vi "TM submodule LSC218.vi"(10 "name (Tmp_M)":string="Tmp_M" caption="Module name", 11 "Super module":T2) -> (0 "Error Out":errorcluster)   [LabVIEW 2021, in "Temperature monitor.lvlib"]
doc: "Magnet module controls: power supply unit (PSU/SMS) and temperature monitor (TM/LSC218).\nPSU controls mainly: switch heater and ramping of current which runs throught coil.\nTM controls temperature of switch, coil and cryostat.\nMessage for magnet is a cluster that contains: {(enum) Command , (variant) Data}\nFor simplifieing of documentation, the Command is noted as a name of instruction, and Data is represented by a requered datatype (mostly cluster) name.\nCommands:\nInitialize(Magnet Config Constants) - Sugesstion: Load configuration constants from configuration file.\nSet field (Set field{B, R, cr}) - B-field[T], R-ramp[A/s], cr - custom ramp[bool].\nSwitch mode(mode) - to persistant, or to ramping.\nBlackout() - undone functionality of emergency deenergizing.\nUpdate() - Important! This triggers update of data from instruments. Shoud occure in regular intervals as priority message.\nResponses:\nMagnet initialized ();\nTM revision(temperature monitor revision);\nMagnet init error(error);\nSetting field(Set Field{B, R, cr});\nWarning(string);\nSwitching to(mode);\nUpdate error(error);\nTM update(TM sensors);\nPSU update(PSU data);\nMagnet status();"
uses:
  Temperature monitor.lvlib
  Typedefs/TM_sensors.ctl
  Typedefs/TM_states.ctl
  <userlib>/MatS Libs/MatS Libs.lvlib
  <userlib>/MatS Libs/MatS Mailman/TypeDefs/Mailbox ref.ctl
  Typedefs/TM_status.ctl
  Typedefs/TM_commands.ctl
  <userlib>/MatS Libs/MatS Mailman/TypeDefs/General message.ctl
panel:
  out "Waveform Graph":waveform(dbl)[](graph)
  in  "Disconnect btn":bool
  in  "History s":i32=60 caption="History [s]" min=10 max=3600 step=1
  out "Temperature history":waveform(dbl)[](graph)
  out "Temperature monitor status":T1 caption="Status" {"Last update" format="%<%H:%M:%S\n%y/%m/%d>T"}
  in  "Stop btn":bool
  in  "Connect btn":bool
  out "Temperatures":T3[](array[typedef]) {"Time stamp" format="%<%H:%M:%S\n%Y/%m/%d>T"}
  in  "VISA resource (COM1)":refnum<visa-resource-name>="COM1" caption="Instrument port"
  in  "Update ms":i32=1000
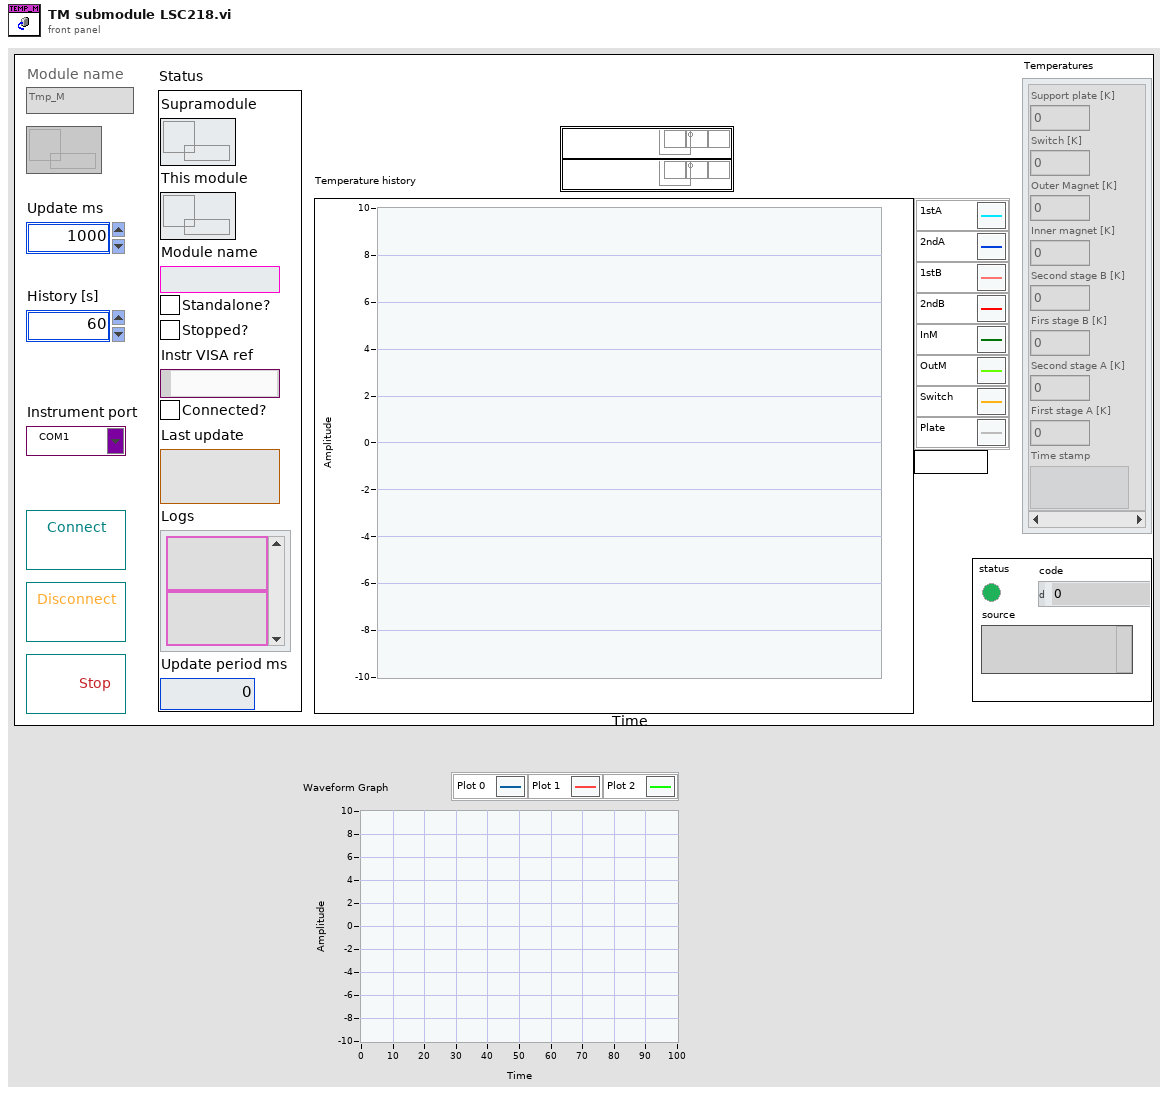
[diagram p1: front panel]
types:
  T1 = typedef "Temperature monitor.lvlib/TM_status.ctl" = cluster{"Supramodule":T2, "This module":T2, "Module name":string, "Standalone?":bool, "Stopped?":bool, "Instr VISA ref":refnum<visa-resource-name>, "Connected?":bool, "Last update":timestamp, "Logs":string[], "Update period ms":u32}
  T2 = typedef "MatS Libs.lvlib/Mailbox ref.ctl" = refnum<queue>
  T3 = typedef "Temperature monitor.lvlib/TM_sensors.ctl" = cluster{"Support plate [K]":dbl, "Switch [K]":dbl, "Outer Magnet [K]":dbl, "Inner magnet [K]":dbl, "Second stage B [K]":dbl, "Firs stage B [K]":dbl, "Second stage A [K]":dbl, "First stage A [K]":dbl, "Time stamp":timestamp}
  T4 = typedef "Temperature monitor.lvlib/TM_states.ctl" = enum16{"Initialize", "Wait for event", "Check message", "Check changes", "End"}
  T5 = enum32{"Bad", "Idle", "Run top level", "Running"}
  T6 = typedef "Temperature monitor.lvlib/TM_commands.ctl" = enum16{"Ignore", "Log", "Connect", "Set timeout", "Update", "Disconnect", "End"}
  T7 = typedef "MatS Libs.lvlib/General message.ctl" = cluster{"Sender":string, "Recipient":string, "Topic":variant, "Content":variant, "Time Stamp":timestamp}
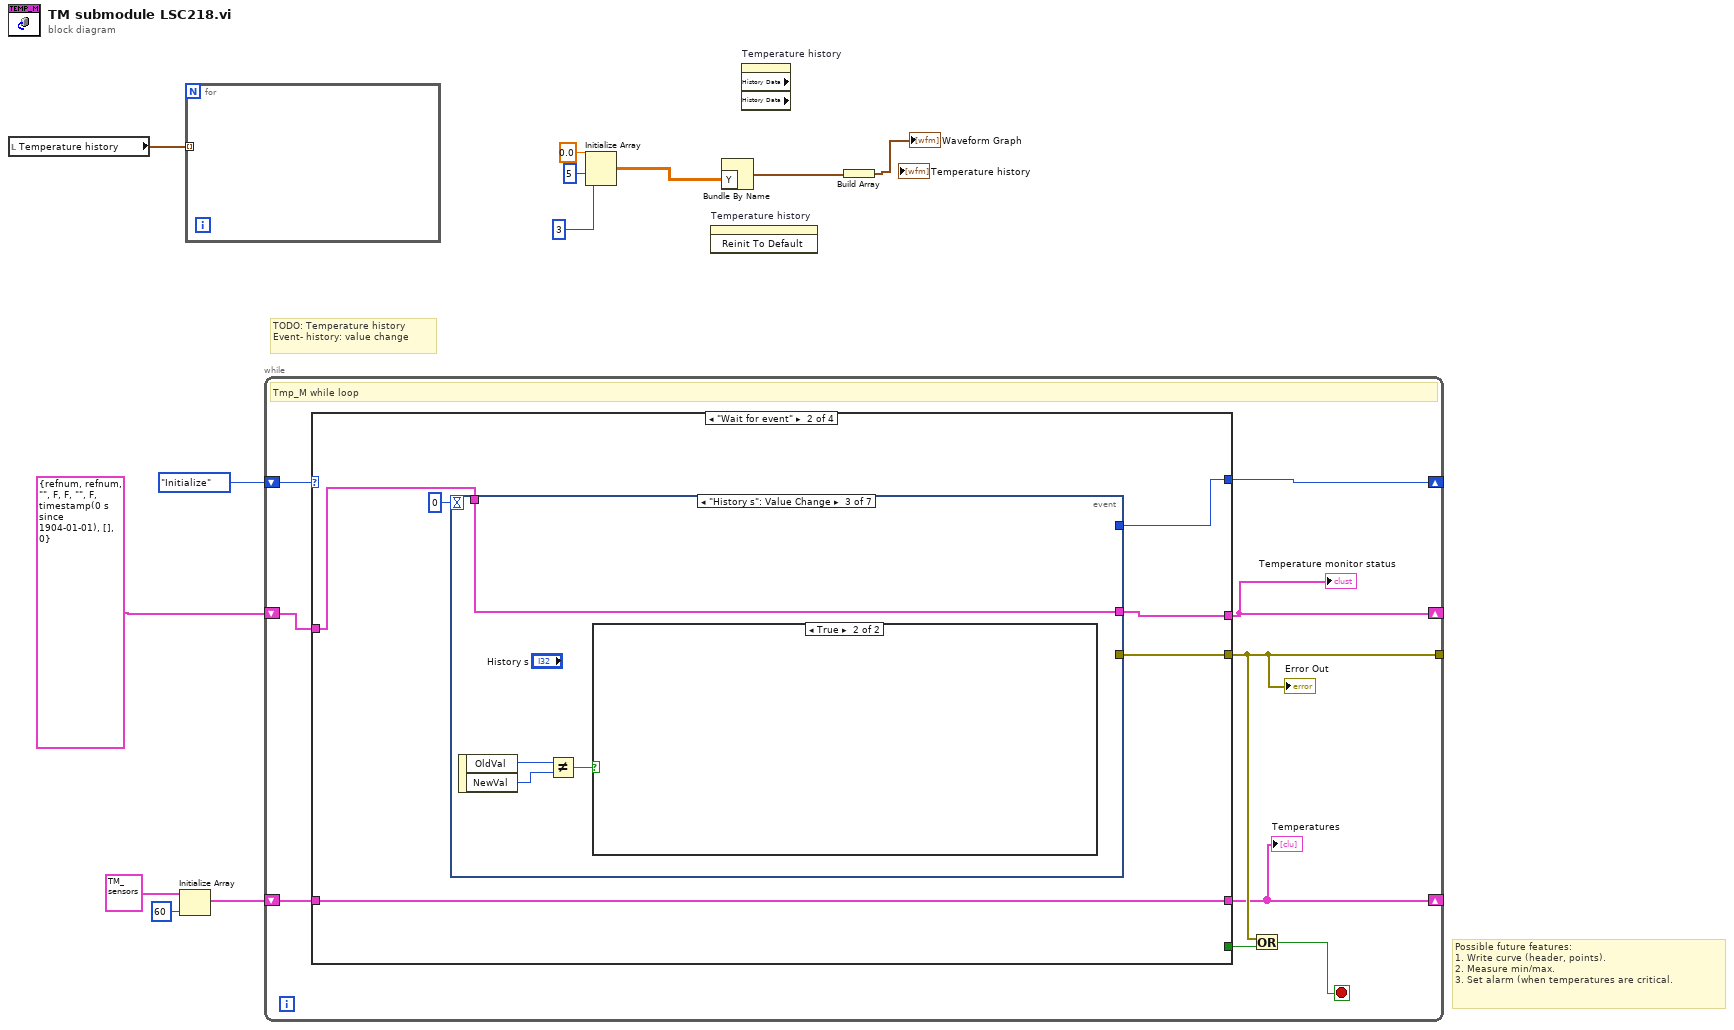
[diagram p0: block diagram]
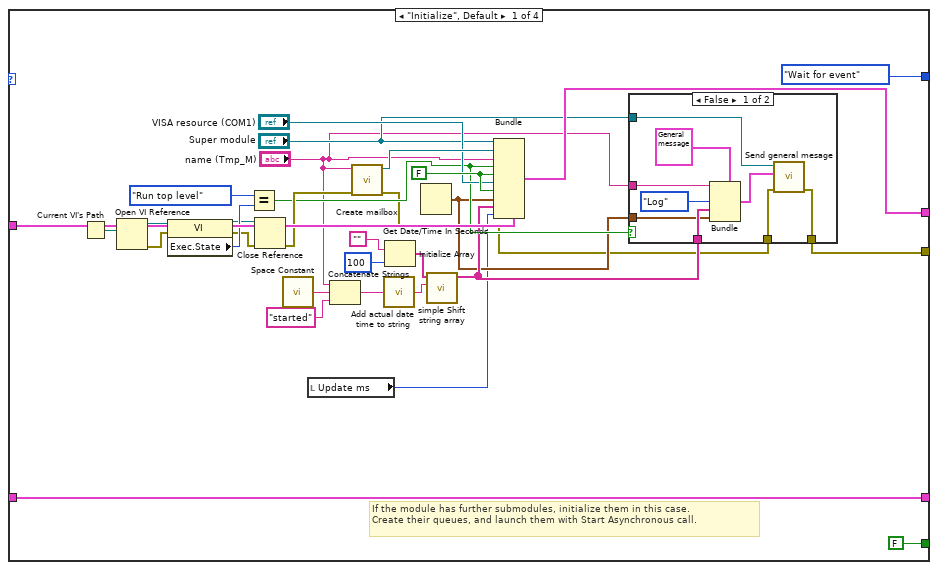
[diagram p2: hidden frame]
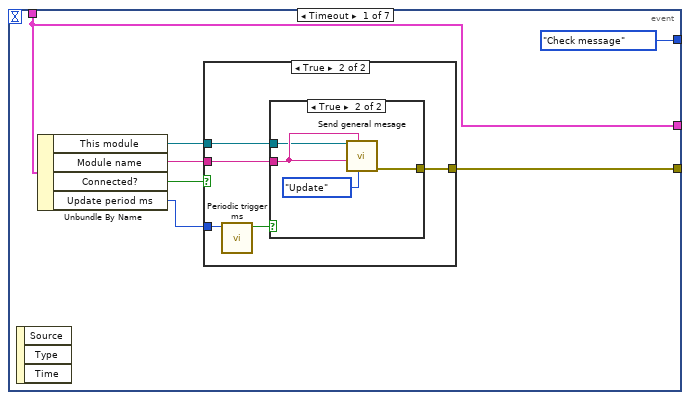
[diagram p4: hidden frame]
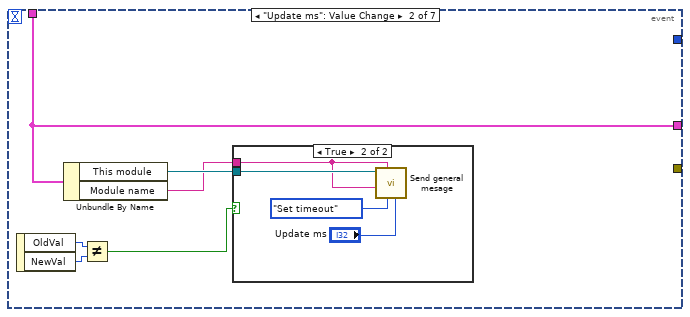
[diagram p7: hidden frame]
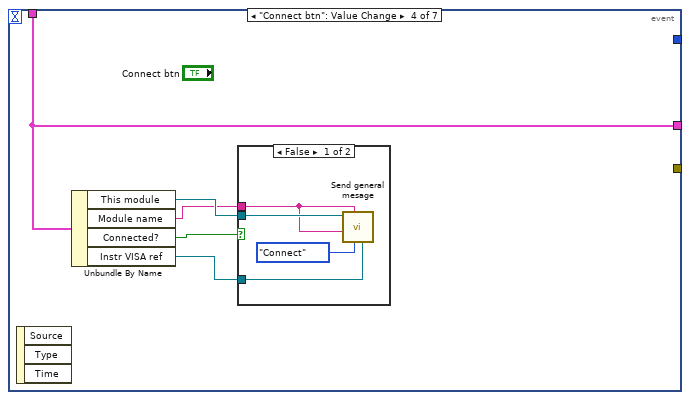
[diagram p10: hidden frame]
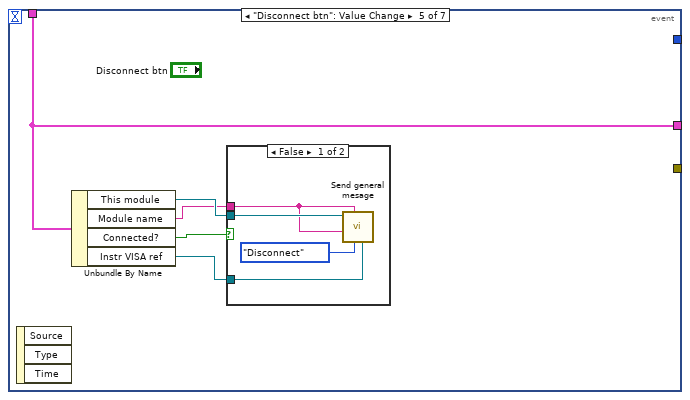
[diagram p12: hidden frame]
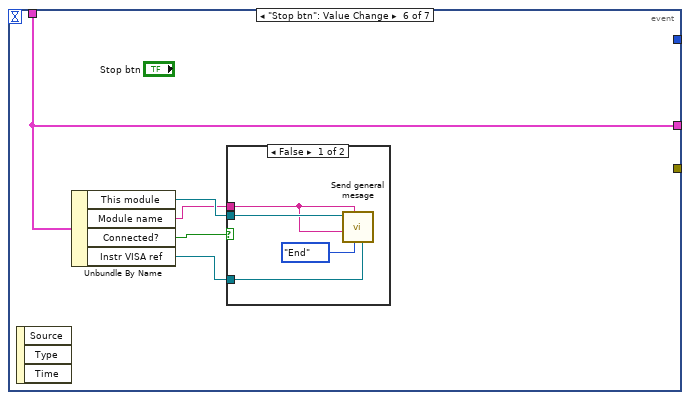
[diagram p14: hidden frame]
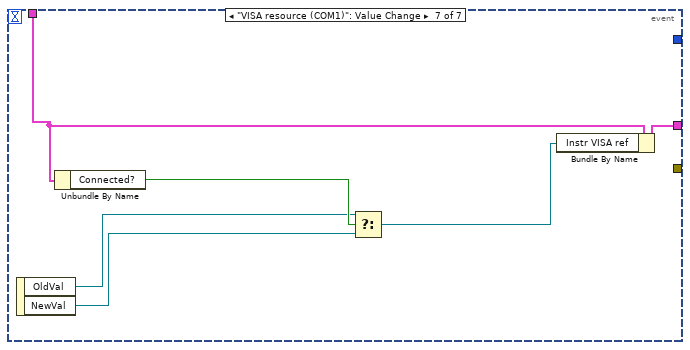
[diagram p16: hidden frame]
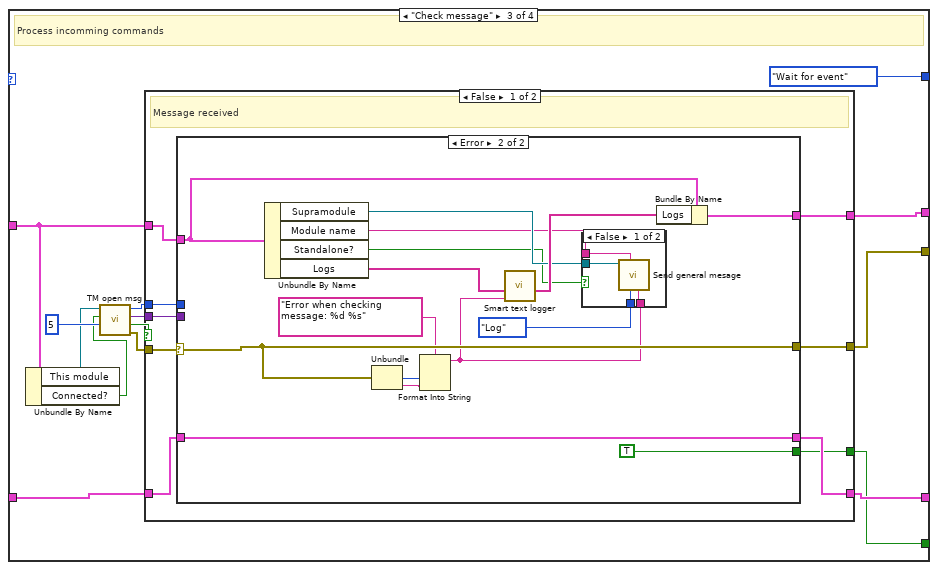
[diagram p17: hidden frame]
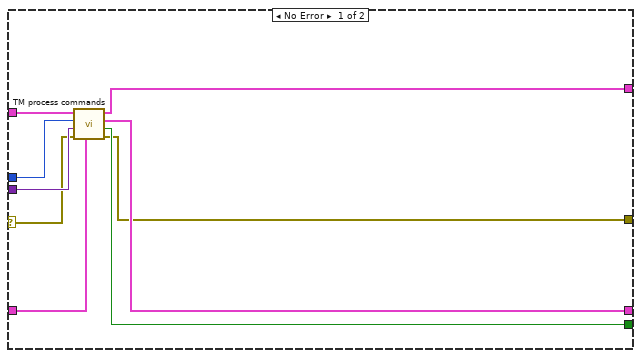
[diagram p18: hidden frame]
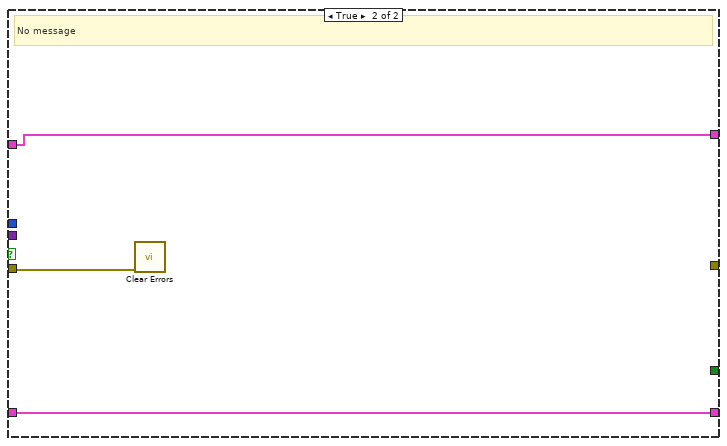
[diagram p20: hidden frame]
diagram:
  # "TODO: Temperature history\nEvent- history: value change"
  # "Possible future features:\n1. Write curve (header, points).\n2. Measure min/max.\n3. Set alarm (when temperatures are critical."
  n1 = local read "Temperature history"() -> (w7:waveform(dbl)[])
  n2 = Initialize Array(T3 {"Support plate [K]"=0.0, "Switch [K]"=0.0, "Outer Magnet [K]"=0.0, "Inner magnet [K]"=0.0, "Second stage B [K]"=0.0, "Firs stage B [K]"=0.0, "Second stage A [K]"=0.0, "First stage A [K]"=0.0, "Time stamp"=timestamp(0 s since 1904-01-01)} ("LSC218 sensors"), 60 ("dimension size")) -> (w12:T3[])
  n3 = for {
    tunnel: w7 -> [_] mode=indexing
  }
  n4 = while {
    shift-right: [w13] -> _
    shift-left: w12 -> [w21]
    tunnel: [w15] -> _
    shift-right: [w18] -> _
    shift-left: TM_states."Initialize" -> [w19]
    shift-right: [w14] -> _
    shift-left: T1 {"Supramodule"=refnum, "This module"=refnum, "Module name"="", "Standalone?"=FALSE, "Stopped?"=FALSE, "Instr VISA ref"="", "Connected?"=FALSE, "Last update"=timestamp(0 s since 1904-01-01), "Logs"=[], "Update period ms"=0} ("Temperature monitor status") -> [w17]
    stop <- w16 stop-if-true
    # "Tmp_M while loop"
    n5 = case shown="\"Wait for event\"" w19 {
      tunnel: w21 -> [w44 w66 w145 w186]
      tunnel: [w44 w66 w144 w186] -> w13
      tunnel: [FALSE _ w140 _] -> w20
      tunnel: [w23 w65 w139 _] -> w15
      tunnel: [TM_states."Wait for event" w68 TM_states."Wait for event" TM_states."End"] -> w18
      tunnel: w17 -> [w47 w63 w132 w187]
      tunnel: [w45 w64 w135 w187] -> w14
      frame "Initialize", Default {
        w43 = FALSE ("Connected?")
        # "If the module has further submodules, initialize them in this case.\nCreate their queues, and launch them with Start Asynchronous call."
        n6 = Current VI's Path() -> (path=w50:path)
        n7 = Open VI Reference(vi path=w50) -> (vi reference=w51:refnum<vi>, error out=w49:errorcluster)  [unwired: 5 in]
        n8 = property class="VI"(reference=w51, error in=w49) -> (reference out=w33:refnum<vi>, error out=w32:errorcluster, "Exec.State"=w35:T5)
        n9 = Equal?(x=T5."Run top level" ("y"), y=w35) -> (x = y?=w29:bool)
        n10 = Close Reference(reference=w33, error in (no error)=w32) -> (error out=w31:errorcluster)
        n11 = call <vilib>:"Space Constant.vi"() -> ("String"=w41:string)
        n12 = local read "Update ms"() -> (w22:i32)
        n13 = Concatenate Strings("name (Tmp_M)", w41, "started") -> (w40:string)
        n14 = call <userlib>:"Create mailbox.vi"("error in (no error)"=w31, "name (unnamed)"="name (Tmp_M)") -> ("error out"=w24:errorcluster, "Mailbox ref"=w46:T2)  [unwired: 3 in, 1 out]
        n15 = call <userlib>:"Add actual date time to string.vi"("String in"=w40) -> ("String out"=w30:string)  [unwired: 4 in]
        n16 = Initialize Array("", 100 ("dimension size")) -> (w36:string[])
        n17 = Get Date/Time In Seconds() -> (seconds since 1Jan1904=w26:timestamp)
        n18 = call <userlib>:"simple Shift string array.vi"("Element in"=w30, "Array in"=w36) -> ("Array out"=w27:string[])  [unwired: 8 in, 1 out]
        n19 = Bundle(cluster=w47, "Supramodule"="Super module", "This module"=w46, "Module name"="name (Tmp_M)", "Standalone?"=w29, "Stopped?"=w43, "Instr VISA ref"="VISA resource (COM1)", "Connected?"=w43, "Last update"=w26, "Logs"=w27, "Update period ms"=w22) -> (w45:T1)
        n20 = case shown="False" w29 {
          tunnel: "Super module" -> [w61 _]
          tunnel: w27 -> [w59 _]
          tunnel: w26 -> [w58 _]
          tunnel: "name (Tmp_M)" -> [w56 _]
          tunnel: w24 -> [w55 w62]
          tunnel: [w54 w62] -> w23
          frame False {
            n21 = Bundle(cluster=T7 {"Sender"="", "Recipient"="", "Topic"=variant(string ""), "Content"=variant, "Time Stamp"=timestamp(0 s since 1904-01-01)} ("Message"), "Sender"=w56, "Topic"=TM_commands."Log" ("Command"), "Content"=w59, "Time Stamp"=w58) -> (w57:T7)  [unwired: 1 in]
            n22 = call <userlib>:"Send general mesage.vi"("error in (no error)"=w55, "Message"=w57, "Mailbox ref in"=w61) -> ("error out"=w54:errorcluster)  [unwired: 6 in, 2 out]
          }
          frame True {
          }
        }
      }
      frame "Wait for event" {
        n23 = event shown="[2] \"History s\": Value Change" {
          selector: _ -> [_ _ _ _ _ _ _]
          dyn-events: _ -> [_ _ _ _ _ _ _]
          timeout: 0 -> [_ _ _ _ _ _ _]
          tunnel: [TM_states."Check message" _ _ _ _ _ _] -> w68
          tunnel: [w74 _ _ _ _ _ _] -> w65
          tunnel: w63 -> [w72 w90 w98 w103 w112 w121 w131]
          tunnel: [w72 w90 w98 w103 w112 w121 w130] -> w64
          event Timeout {
            n24 = event-data() -> ()  [unwired: 1 in, 3 out]
            n25 = Unbundle By Name(w72) -> ("This module"=w70:T2, "Module name"=w71:string, "Connected?"=w73:bool, "Update period ms"=w69:u32)
            n26 = case shown="True" w73 {
              tunnel: w69 -> [_ w80]
              tunnel: [_ w79] -> w74
              tunnel: w71 -> [_ w77]
              tunnel: w70 -> [_ w76]
              frame False {
              }
              frame True {
                n27 = call <userlib>:"Periodic trigger ms.vi"("Period ms"=w80) -> ("Trigger"=w78:bool)  [unwired: 6 in]
                n28 = case shown="True" w78 {
                  tunnel: [_ w84] -> w79
                  tunnel: w77 -> [_ w83]
                  tunnel: w76 -> [_ w82]
                  frame False {
                  }
                  frame True {
                    n29 = call <userlib>:"Send general mesage.vi"("Topic"=TM_commands."Update" ("Command"), "Sender"=w83, "Recipient"=w83, "Mailbox ref in"=w82) -> ("error out"=w84:errorcluster)  [unwired: 5 in, 2 out]
                  }
                }
              }
            }
          }
          event "Update ms": Value Change {
            n30 = event-data() -> ("OldVal"=w87:i32, "NewVal"=w86:i32)  [unwired: 1 in]
            n31 = Unbundle By Name(w90) -> ("This module"=w89:T2, "Module name"=w88:string)
            n32 = Not Equal?(x=w87, y=w86) -> (x != y?=w85:bool)
            n33 = case shown="True" w85 {
              tunnel: w89 -> [_ w94]
              tunnel: w88 -> [_ w93]
              frame False {
              }
              frame True {
                n34 = call <userlib>:"Send general mesage.vi"("Content"="Update ms", "Topic"=TM_commands."Set timeout" ("Command"), "Sender"=w93, "Recipient"=w93, "Mailbox ref in"=w94) -> ()  [unwired: 4 in, 3 out]
              }
            }
          }
          event "History s": Value Change {
            n35 = event-data() -> ("OldVal"=w97:i32, "NewVal"=w96:i32)  [unwired: 1 in]
            n36 = Not Equal?(x=w97, y=w96) -> (x != y?=w95:bool)
            n37 = case shown="True" w95 {
              frame False {
              }
              frame True {
              }
            }
          }
          event "Connect btn": Value Change {
            n38 = event-data() -> ()  [unwired: 1 in, 3 out]
            n39 = Unbundle By Name(w103) -> ("This module"=w101:T2, "Module name"=w100:string, "Connected?"=w102:bool, "Instr VISA ref"=w99:refnum<visa-resource-name>)
            n40 = case shown="False" w102 {
              tunnel: w101 -> [w107 _]
              tunnel: w100 -> [w106 _]
              tunnel: w99 -> [w104 _]
              frame False {
                n41 = call <userlib>:"Send general mesage.vi"("Content"=w104, "Topic"=TM_commands."Connect" ("Command"), "Sender"=w106, "Recipient"=w106, "Mailbox ref in"=w107) -> ()  [unwired: 4 in, 3 out]
              }
              frame True {
              }
            }
          }
          event "Disconnect btn": Value Change {
            n42 = event-data() -> ()  [unwired: 1 in, 3 out]
            n43 = Unbundle By Name(w112) -> ("This module"=w110:T2, "Module name"=w109:string, "Connected?"=w111:bool, "Instr VISA ref"=w108:refnum<visa-resource-name>)
            n44 = case shown="False" w111 {
              tunnel: w110 -> [w116 _]
              tunnel: w109 -> [w115 _]
              tunnel: w108 -> [w113 _]
              frame False {
                n45 = call <userlib>:"Send general mesage.vi"("Content"=w113, "Topic"=TM_commands."Disconnect" ("Command"), "Sender"=w115, "Recipient"=w115, "Mailbox ref in"=w116) -> ()  [unwired: 4 in, 3 out]
              }
              frame True {
              }
            }
          }
          event "Stop btn": Value Change {
            n46 = event-data() -> ()  [unwired: 1 in, 3 out]
            n47 = Unbundle By Name(w121) -> ("This module"=w119:T2, "Module name"=w118:string, "Connected?"=w120:bool, "Instr VISA ref"=w117:refnum<visa-resource-name>)
            n48 = case shown="False" w120 {
              tunnel: w119 -> [w125 _]
              tunnel: w118 -> [w124 _]
              tunnel: w117 -> [w122 _]
              frame False {
                n49 = call <userlib>:"Send general mesage.vi"("Content"=w122, "Topic"=TM_commands."End" ("Command"), "Sender"=w124, "Recipient"=w124, "Mailbox ref in"=w125) -> ()  [unwired: 4 in, 3 out]
              }
              frame True {
              }
            }
          }
          event "VISA resource (COM1)": Value Change {
            n50 = event-data() -> ("OldVal"=w128:refnum<visa-resource-name>, "NewVal"=w127:refnum<visa-resource-name>)  [unwired: 1 in]
            n51 = Unbundle By Name(w131) -> ("Connected?"=w129:bool)
            n52 = Select(t=w128, s=w129, f=w127) -> (s? t:f=w126:refnum<visa-resource-name>)
            n53 = Bundle By Name(cluster=w131, "Instr VISA ref"=w126) -> (w130:T1)
          }
        }
      }
      frame "Check message" {
        # "Process incomming commands"
        n54 = Unbundle By Name(w132) -> ("This module"=w133:T2, "Connected?"=w134:bool)
        n55 = call "TM open msg.vi"("timeout ms (1000)"=5, "Connected"=w134, "Queue in"=w133) -> ("error out"=w142:errorcluster, "timed out?"=w136:bool, "Data"=w141:variant, "Command"=w143:T6)  [unwired: 3 in, 2 out]
        n56 = case shown="False" w136 {
          tunnel: w145 -> [w154 w185]
          tunnel: [w153 w185] -> w144
          tunnel: w143 -> [w152 _]
          tunnel: w142 -> [w151 w184]
          tunnel: w141 -> [w150 _]
          tunnel: [w149 _] -> w140
          tunnel: [w148 _] -> w139
          tunnel: [w147 w183] -> w135
          tunnel: w132 -> [w146 w183]
          frame False {
            # "Message received"
            n57 = case shown="Error" w151 {
              selector: w151 -> [w158 w176]
              tunnel: w152 -> [w155 _]
              tunnel: w154 -> [w163 w178]
              tunnel: [w162 w178] -> w153
              tunnel: [w160 TRUE] -> w149
              tunnel: w150 -> [w161 _]
              tunnel: [w157 w176] -> w148
              tunnel: [w159 w175] -> w147
              tunnel: w146 -> [w156 w168]
              frame No Error {
                n58 = call "TM process commands.vi"("Array in"=w163, "error in (no error)"=w158, "Data"=w161, "Command"=w155, "Temperature monitor status in"=w156) -> ("error out"=w157:errorcluster, "End?"=w160:bool, "Array out"=w162:T3[], "Temperature monitor status out"=w159:T1)  [unwired: 3 in]
              }
              frame Error {
                n59 = Unbundle By Name(w168) -> ("Supramodule"=w172:T2, "Module name"=w170:string, "Standalone?"=w171:bool, "Logs"=w169:string[])
                n60 = Unbundle(w176) -> ("code"=w165:i32, "source"=w166:string)  [unwired: 1 out]
                n61 = Format Into String(format string="Error when checking message: %d %s", w165, w166) -> (resulting string=w164:string)  [unwired: 2 in, 1 out]
                n62 = call <userlib>:"Smart text logger.vi"("Message"=w164, "Logs in"=w169) -> ("Logs out"=w174:string[])  [unwired: 9 in]
                n63 = case shown="False" w171 {
                  tunnel: w172 -> [w182 _]
                  tunnel: w170 -> [w181 _]
                  tunnel: TM_commands."Log" ("Command") -> [w180 _]
                  tunnel: w164 -> [w179 _]
                  frame False {
                    n64 = call <userlib>:"Send general mesage.vi"("Content"=w179, "Topic"=w180, "Sender"=w181, "Mailbox ref in"=w182) -> ()  [unwired: 5 in, 3 out]
                  }
                  frame True {
                  }
                }
                n65 = Bundle By Name(cluster=w168, "Logs"=w174) -> (w175:T1)
              }
            }
          }
          frame True {
            # "No message"
            n66 = call <vilib>:"Clear Errors.vi"("error in (no error)"=w184) -> ()  [unwired: 5 in, 2 out]
          }
        }
      }
      frame "End" {
      }
    }
    "Error Out" <- w15
    "Temperatures" <- w13
    "Temperature monitor status" <- w14
    n67 = Or(x=w15, y=w20) -> (x .or. y?=w16:bool)
  }
  n68 = Initialize Array(0.0 ("element"), 5 ("dimension size"), 3 ("dimension size")) -> (w1:dbl[][])
  n69 = invoke on="Temperature history" class="WFChart (strict)" method="Reinit To Default"() -> ()  [unwired: 3 in, 3 out]
  n70 = Bundle By Name("Y"=w1) -> (w6:waveform(dbl))  [unwired: 1 in]
  n71 = property on="Temperature history" class="WFChart (strict)" props=["History Data", "History Data"]() -> ()  [unwired: 2 in, 4 out]
  n72 = Build Array(w6) -> (→"Waveform Graph":waveform(dbl)[])
